vi "Start Task.vi"(8 "error in (no error)":errorcluster, 11 "DAQ Actor (Slave) in":refnum<class "DAQ Actor (Slave).lvclass">) -> (0 "error out":errorcluster, 3 "DAQ Actor (Slave) out":refnum<class "DAQ Actor (Slave).lvclass">)   [LabVIEW 2018, in "Data Acquisition.lvlib" / "DAQ Actor (Slave).lvclass"]
uses:
  DAQ Actor (Slave).lvclass
  DAQ Actor (Slave).lvclass/DAQ Actor (Slave).ctl
  <vilib>/ActorFramework/Message Enqueuer/Message Enqueuer.lvclass/Message Enqueuer.ctl
  <vilib>/ActorFramework/Message Enqueuer/Enqueue.vi
  DAQ Actor Messages/Start Task Msg/Start Task Msg.lvclass
  C:/Program Files (x86)/National Instruments/LabVIEW 2018/vi.lib/ActorFramework/Message/Message.lvclass
  <vilib>/ActorFramework/Message Priority Queue/Priority Enqueue.vi
  Class DAQ Actor/DAQ Actor.lvclass
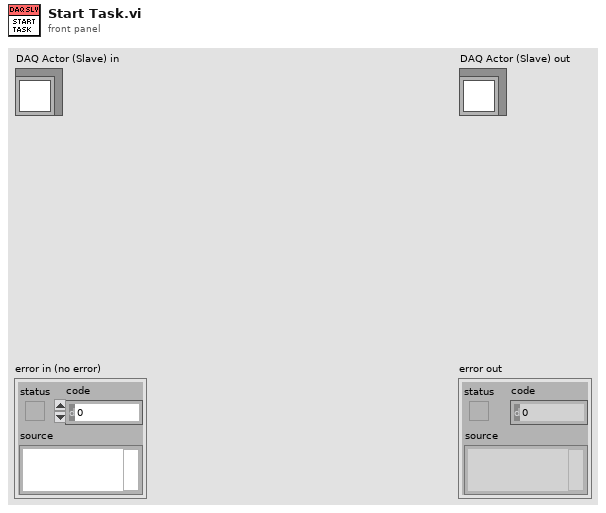
[diagram p1: front panel]
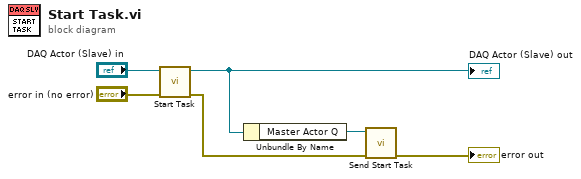
[diagram p0: block diagram]
diagram:
  n1 = call-parent "Start Task.vi"("error in (no error)"="error in (no error)", "DAQ Actor in"="DAQ Actor (Slave) in") -> ("error out"=w2:errorcluster, "DAQ Actor out"=w4:refnum<class "DAQ Actor (Slave).lvclass">)  [unwired: 8 in]
  "DAQ Actor (Slave) out" <- w4
  n2 = Unbundle By Name(w4) -> ("Master Actor Q"=w3:refnum<class "Message Enqueuer.lvclass">)
  n3 = call "Send Start Task.vi"("error in (no error)"=w2, "Message Enqueuer"=w3) -> ("error out"=→"error out":errorcluster)  [unwired: 8 in, 1 out]
